vi "test Parse DBL Array2.vi"(11 "Test Case In":refnum<class "Test Simple CSV Parser.lvclass">) -> (0 "error out":errorcluster, 3 "Test Case Out":refnum<class "Test Simple CSV Parser.lvclass">)   [LabVIEW 2024, in "Test Simple CSV Parser.lvclass"]
uses:
  Test Simple CSV Parser.lvclass
  C:/Program Files/National Instruments/LabVIEW 2025/vi.lib/Astemes/LUnit/Test Case.lvclass
  CSV Parser/Simple CSV Parser/Simple CSV Parser.lvclass
  <vilib>/Astemes/LUnit/Test Case.lvclass/Test Case.ctl
  <vilib>/Astemes/LUnit/Append Fail Result.vi
  <vilib>/Astemes/LUnit/Append Pass Result.vi
  <vilib>/Astemes/LUnit/Run In UI.vi
  <vilib>/Astemes/LUnit/Test Case.lvclass
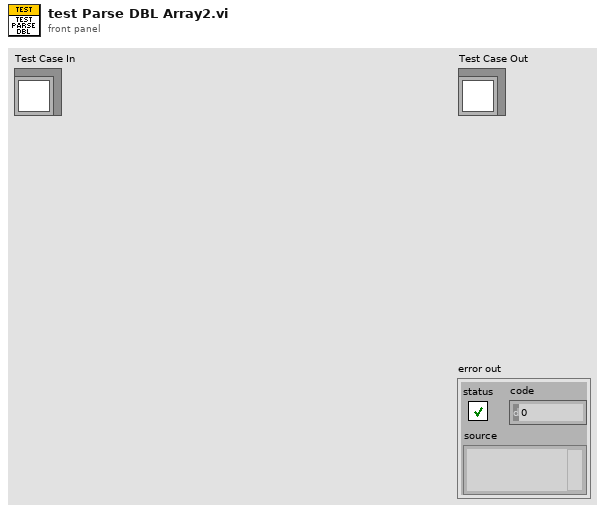
[diagram p1: front panel]
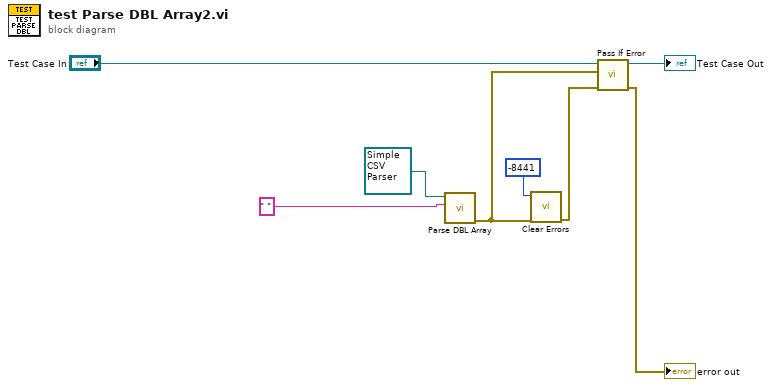
[diagram p0: block diagram]
diagram:
  n1 = call-dynamic "Parse DBL Array.vi"("csv string"=" ", "Simple CSV Parser in"=refnum<class "Simple CSV Parser.lvclass"> refnum) -> ("error out"=w2:errorcluster)  [unwired: 7 in, 2 out]
  n2 = call <vilib>:"Clear Errors.vi"("error in (no error)"=w2, "specific error code to clear (0: all)"=-8441) -> ("error out"=w1:errorcluster)  [unwired: 4 in, 1 out]
  n3 = call <vilib>:"Pass If Error.vi"("error in (no error)"=w1, "Assert error"=w2, "LUnit Test Case In"="Test Case In") -> ("error out"=→"error out":errorcluster, "LUnit Test Case Out"=→"Test Case Out":refnum<class "Test Simple CSV Parser.lvclass">)  [unwired: 7 in]
